vi "checkValues.vi"(8 "error in (no error)":errorcluster, 11 "ScanCreator in":refnum<class "ScanCreator.lvclass">) -> (0 "error out":errorcluster, 2 "passed":bool, 3 "ScanCreator out":refnum<class "ScanCreator.lvclass">)   [LabVIEW 2011, in "Views.lvlib" / "ScriptEditor.lvlib" / "ScanCreator.lvclass"]
uses:
  ScanCreator.lvclass
  ScanCreator.lvclass/ScanCreator.ctl
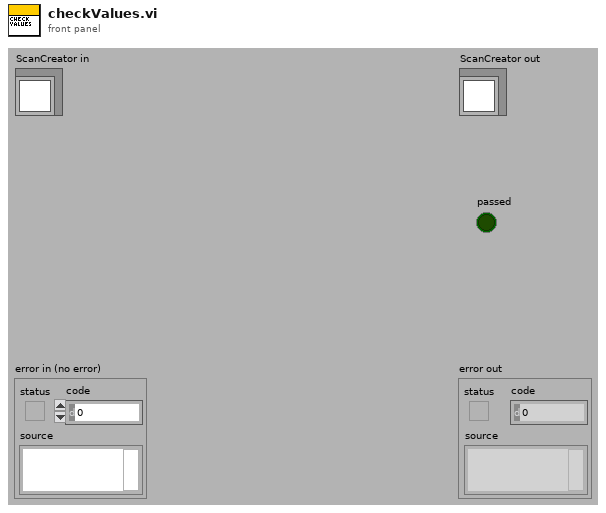
[diagram p1: front panel]
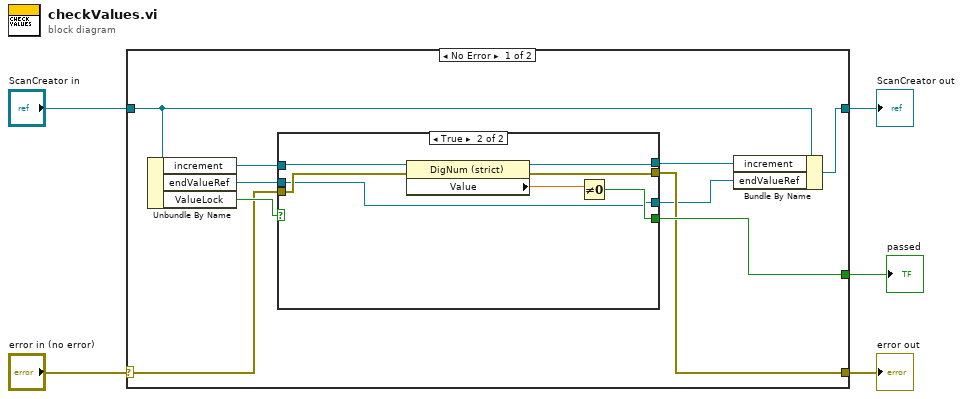
[diagram p0: block diagram]
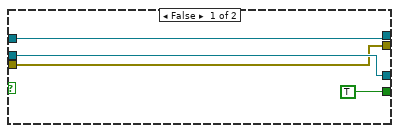
[diagram p2: hidden frame]
diagram:
  n1 = case shown="No Error" "error in (no error)" {
    selector: "error in (no error)" -> [w12 w28]
    tunnel: [w10 w28] -> w4
    tunnel: [w6 w27] -> w2
    tunnel: "ScanCreator in" -> [w9 w27]
    tunnel: [w11 _] -> w1
    frame No Error {
      n2 = Unbundle By Name(w9) -> ("increment"=w14:refnum<vi>, "endValueRef"=w13:refnum<vi>, "ValueLock"=w15:bool)
      n3 = case shown="True" w15 {
        tunnel: w14 -> [w18 w26]
        tunnel: w13 -> [w19 w20]
        tunnel: w12 -> [w17 w22]
        tunnel: [TRUE w21] -> w11
        tunnel: [w17 w24] -> w10
        tunnel: [w18 w23] -> w8
        tunnel: [w19 w20] -> w7
        frame False {
        }
        frame True {
          n4 = property class="DigNum (strict)"(reference=w26, error in=w22) -> (reference out=w23:refnum<vi>, error out=w24:errorcluster, "Value"=w25:dbl)
          n5 = Not Equal To 0?(x=w25) -> (x != 0?=w21:bool)
        }
      }
      n6 = Bundle By Name(cluster=w9, "increment"=w8, "endValueRef"=w7) -> (w6:refnum<class "ScanCreator.lvclass">)
    }
    frame Error {
    }
  }
  "error out" <- w4
  "ScanCreator out" <- w2
  "passed" <- w1
